vi "Update Data Buffer.vi"(6 "gain":dbl, 8 "error in (no error)":errorcluster, 9 "dt":dbl, 10 "Data Buffer":T1, 11 "Calculation Worker in":refnum<class "Calculation Worker.lvclass">) -> (0 "error out":errorcluster, 3 "Calculation Worker out":refnum<class "Calculation Worker.lvclass">)   [LabVIEW 2020, in "Calculation Worker.lvlib" / "Calculation Worker.lvclass"]
uses:
  Calculation Worker.lvclass
  GPU FFT Calculator/GPU FFT Calculator/Data Source Buffer.ctl
  Calculation Worker.lvclass/Calculation Worker.ctl
  Data Source/Data Source/Data Source.lvclass
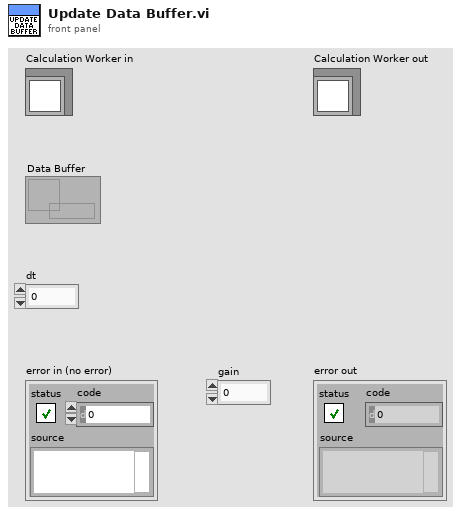
[diagram p1: front panel]
types:
  T1 = typedef "Data Source.lvlib/Data Source.lvclass/Data Source Buffer.ctl" = refnum<data-value>
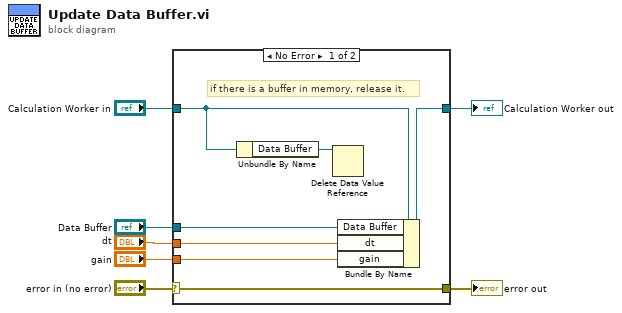
[diagram p0: block diagram]
diagram:
  n1 = case shown="No Error" "error in (no error)" {
    selector: "error in (no error)" -> [w12 w16]
    tunnel: [w12 w16] -> w6
    tunnel: [w11 w15] -> w4
    tunnel: "Calculation Worker in" -> [w14 w15]
    tunnel: "Data Buffer" -> [w10 _]
    tunnel: "dt" -> [w9 _]
    tunnel: "gain" -> [w8 _]
    frame No Error {
      # "if there is a buffer in memory, release it."
      n2 = Unbundle By Name(w14) -> ("Data Buffer"=w13:T1)
      n3 = Delete Data Value Reference(data value reference=w13) -> ()  [unwired: 1 in, 2 out]
      n4 = Bundle By Name(cluster=w14, "Data Buffer"=w10, "dt"=w9, "gain"=w8) -> (w11:refnum<class "Calculation Worker.lvclass">)
    }
    frame Error {
    }
  }
  "error out" <- w6
  "Calculation Worker out" <- w4
